vi "CleanUp.vi"(8 "error in (no error)":errorcluster, 11 "reference in":refnum<class "TestCSMSuite.lvclass">) -> (0 "error out":errorcluster, 3 "reference out":refnum<class "TestCSMSuite.lvclass">)   [LabVIEW 2017, in "TestCSMSuite.lvclass"]
uses:
  TestCSMSuite.lvclass
  <vilib>/addons/_JKI Toolkits/VI Tester/TestSuite.llb/TestSuite.lvclass
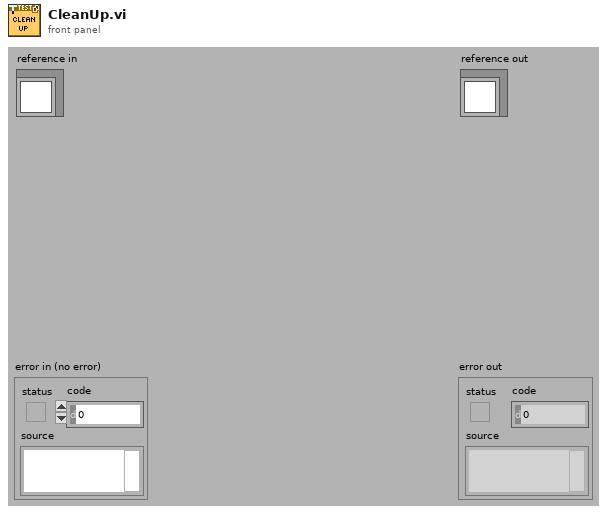
[diagram p1: front panel]
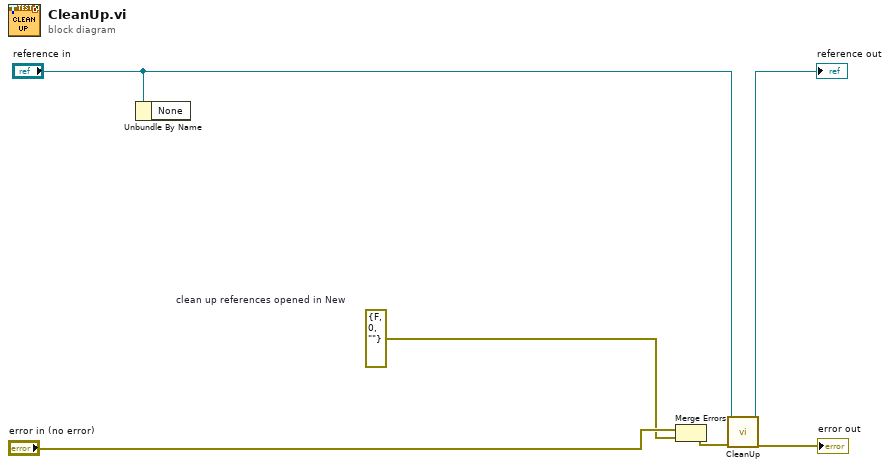
[diagram p0: block diagram]
diagram:
  w5 = errorcluster {"status"=FALSE, "code"=0, "source"=""}  # clean up references opened in New
  n1 = Unbundle By Name("reference in") -> ()  [unwired: 1 out]
  n2 = Merge Errors("error in (no error)", w5) -> (w2:errorcluster)
  n3 = call-parent "CleanUp.vi"("error in (no error)"=w2, "TestSuite in"="reference in") -> ("error out"=→"error out":errorcluster, "TestSuite out"=→"reference out":refnum<class "TestCSMSuite.lvclass">)  [unwired: 8 in]
